vi "LVClass_WavefrontCorrector Check User Preferences.vi"(0 "WavefrontCorrector in":refnum<class "WavefrontCorrector.lvclass">, 5 "Mirror preferences":T1, 11 "error in (no error)":errorcluster) -> (4 "WavefrontCorrector out":refnum<class "WavefrontCorrector.lvclass">, 15 "error out":errorcluster)   [LabVIEW 2020, in "WavefrontCorrector.lvclass"]
doc: "Assert requested preferences fulfill specifications constraints.\n\n--------------------------------------------------------------------------------\n\n<B>correctorIn </B> : WavefrontCorrector object.\n<B>correctorOut </B> : WavefrontCorrector object.\n<B>sleep_after_movement </B> : WavefrontCorrector preferences : Time to stabilization (ms).\n<B>min </B> : WavefrontCorrector preferences : lowest command value.\n<B>max </B> : WavefrontCorrector preferences : highest command value.\n<B>validity </B> : WavefrontCorrector preferences : status.\n<B>fixed_values </B> : WavefrontCorrector preferences : fixed positions.\n<B>ErrorIn </B> : Error\n<B>ErrorOut </B> : Error\n\n--------------------------------------------------------------------------------"
uses:
  WavefrontCorrector.lvclass
  Wavefront Corrector states.ctl
  Wavefront Corrector states - ONE.ctl
  WavefrontCorrector.lvclass/WavefrontCorrector.ctl
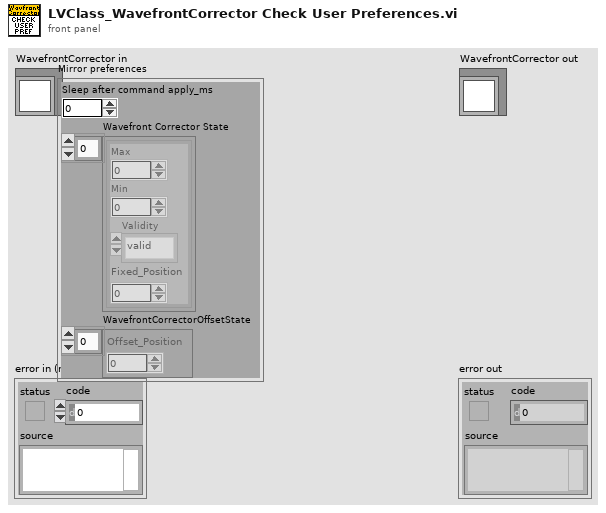
[diagram p1: front panel]
types:
  T1 = typedef "Wavefront Corrector states.ctl" = cluster{"Sleep after command apply_ms":i32, "Wavefront Corrector State":T2[], "WavefrontCorrectorOffsetState":sgl[]}
  T2 = typedef "Wavefront Corrector states - ONE.ctl" = cluster{"Max":sgl, "Min":sgl, "Validity":enum16{"valid", "fixed", "invalid"}, "Fixed_Position":sgl}
  T3 = typedef "ClassID.ctl" = i64
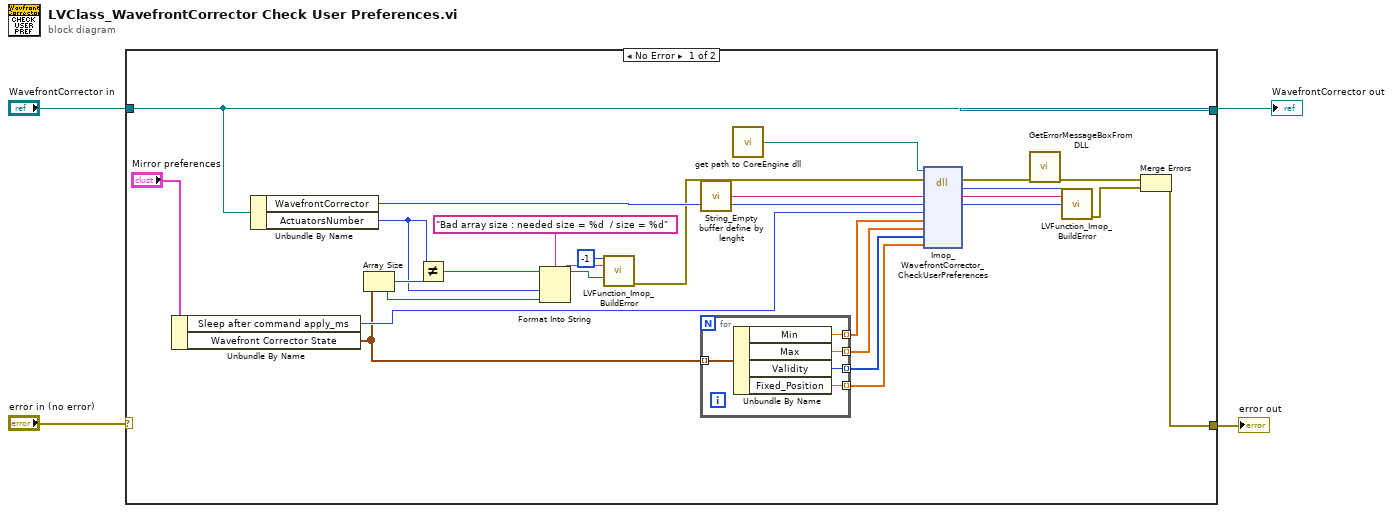
[diagram p0: block diagram]
diagram:
  n1 = case shown="No Error" "error in (no error)" {
    selector: "error in (no error)" -> [_ w36]
    tunnel: [w27 w36] -> w1
    tunnel: [w26 w35] -> w2
    tunnel: "WavefrontCorrector in" -> [w26 w35]
    frame No Error {
      n2 = Unbundle By Name("Mirror preferences") -> ("Sleep after command apply_ms"=w20:i32, "Wavefront Corrector State"=w19:T2[])
      n3 = Unbundle By Name(w26) -> ("WavefrontCorrector"=w25:T3, "ActuatorsNumber"=w15:i32)
      n4 = Array Size(array=w19) -> (size(s)=w16:i32)
      n5 = Not Equal?(x=w15, y=w16) -> (x != y?=w10:bool)
      n6 = Format Into String(format string="Bad array size : needed size = %d  / size = %d" ("String to Prepend to source (\"\")"), w15, w16) -> (resulting string=w17:string)  [unwired: 2 in, 1 out]
      n7 = call "LVFunction_Imop_BuildError.vi"("code"=-1, "String to Prepend to source (\"\")"=w17, "Activate error? (true)"=w10) -> ("error out"=w8:errorcluster)  [unwired: 12 in]
      n8 = call "String_Empty buffer define by lenght.vi"() -> ("Empty buffer"=w13:string)  [unwired: 1 in]
      n9 = for {
        tunnel: w19 -> [w34] mode=indexing
        tunnel: [w33] -> w7 mode=indexing
        tunnel: [w32] -> w6 mode=indexing
        tunnel: [w31] -> w12 mode=indexing
        tunnel: [w30] -> w11 mode=indexing
        n10 = Unbundle By Name(w34) -> ("Min"=w33:sgl, "Max"=w32:sgl, "Validity"=w31:enum16{"valid", "fixed", "invalid"}, "Fixed_Position"=w30:sgl)
      }
      n11 = call "get path to CoreEngine dll.vi"() -> ("path to wavekit library"=w14:path)  [unwired: 14 in, 1 out]
      n12 = dll-call lib="D:/SOFTware/HASO_v3/SVN_trunk/ImOpCoreEngine4_LV2011/DLLs/c_interface_vc100.dll" fn="Imop_WavefrontCorrector_CheckUserPreferences"(path in=w14, error in=w8, "message"=w13, "WavefrontCorrection"=w25, "sleep_after_movement"=w20, "min"=w7, "max"=w6, "validity"=w12, "fixed_value"=w11) -> (error out=w24:errorcluster, "return type"=w23:i32, "message"=w22:string, "WavefrontCorrection"=w5:i64)  [unwired: 6 in, 1 out]
      n13 = call "GetErrorMessageBoxFromDLL.vi"("error IN"=w24) -> ("error OUT"=w29:errorcluster)  [unwired: 10 in]
      n14 = call "LVFunction_Imop_BuildError.vi"("code"=w23, "String to Prepend to source (\"\")"=w22, "Adresse"=w5) -> ("error out"=w28:errorcluster)  [unwired: 12 in]
      n15 = Merge Errors(w29, w28) -> (w27:errorcluster)
    }
    frame Error {
    }
  }
  "error out" <- w1
  "WavefrontCorrector out" <- w2
